vi "Actor Core.vi"(8 "error in":errorcluster, 11 "Island in":refnum<class "Island.lvclass">) -> (0 "error out":errorcluster, 3 "Actor out":refnum<class "Actor.lvclass">)   [LabVIEW 2018, in "Island Actor.lvlib" / "Island.lvclass"]
doc: "(<B>Filename</B>: Actor Framework.lvlib:Actor.lvclass:Actor Core.vi)\n\nReceives messages to the actor, reacts to them, and initiates any error handling that may shut the actor down.\n\nDescendant classes may override this VI to append parallel tasks for the actor to complete while it handles messages. Overrides use the Call Parent Method node."
uses:
  Island.lvclass
  C:/Users/Administrator/Desktop/LabVIEW EMS/EMS Generic Actor/EMS Generic/EMS Generic.lvclass
  C:/Users/Administrator/Desktop/LabVIEW EMS/Device Communication and Control Abstract Actor/Device Communication and Control Abstract/Device Communication and Control Abstract.lvclass
  C:/Users/Administrator/Desktop/LabVIEW EMS/Optimization/Generic Optimization Actor/Generic Optimization/Generic Optimization.lvclass
  <vilib>/ActorFramework/Actor/Actor.lvclass
  EMS Generic Actor/EMS Generic/EMS Generic.lvclass/EMS Generic.ctl
  <vilib>/ORNL/CSEISMIC DDS/CSEISMIC DDS Base/Data Types/DER_VF.ctl
  <vilib>/ORNL/CSEISMIC DDS/CSEISMIC DDS Base/Data Types/Controls/DeviceID.ctl
  <vilib>/ActorFramework/Actor/Actor.lvclass/Actor.ctl
  Device Communication and Control Abstract Actor/Device Communication and Control Abstract/Device Communication and Control Abstract.lvclass/Device Communication and Control Abstract.ctl
  Device Communication and Control Abstract Actor/Device Communication and Control Abstract Messages/Set DER VF Msg/Set DER VF Msg.lvclass/Set DER VF Msg.ctl
  <vilib>/ActorFramework/Message Enqueuer/Message Enqueuer.lvclass/Message Enqueuer.ctl
  Generic Optimization Actor/Generic Optimization/Optimization Controls/PCC Data.ctl
  <vilib>/ORNL/CSEISMIC DDS/CSEISMIC DDS Base/Data Types/SmartRelay_Measurement.ctl
  <vilib>/ORNL/CSEISMIC DDS/CSEISMIC DDS Base/Data Types/PCC_Transition.ctl
  Device Communication and Control Abstract Actor/Device Communication and Control Abstract Messages/Set PCC Transition Msg/Set PCC Transition Msg.lvclass/Set PCC Transition Msg.ctl
  Device Communication and Control Abstract Actor/Device Communication and Control Abstract Messages/Set DER VF Msg/Send Set DER VF.vi
  <vilib>/ActorFramework/Actor/Read Caller Enqueuer.vi
  Device Communication and Control Abstract Actor/Device Communication and Control Abstract Messages/Set PCC Transition Msg/Send Set PCC Transition.vi
  <vilib>/ActorFramework/Message Enqueuer/Enqueue.vi
  Device Communication and Control Abstract Actor/Device Communication and Control Abstract/Device Communication and Control Abstract.lvclass
  C:/Program Files (x86)/National Instruments/LabVIEW 2018/vi.lib/ActorFramework/Actor/Actor.lvclass
  Device Communication and Control Abstract Actor/Device Communication and Control Abstract Messages/Set DER VF Msg/Set DER VF Msg.lvclass
  C:/Program Files (x86)/National Instruments/LabVIEW 2018/vi.lib/ActorFramework/Message/Message.lvclass
  Device Communication and Control Abstract Actor/Device Communication and Control Abstract Messages/Set PCC Transition Msg/Set PCC Transition Msg.lvclass
  <vilib>/ActorFramework/Message Priority Queue/Priority Enqueue.vi
  Generic Optimization Actor/Generic Optimization/Generic Optimization.lvclass
  <vilib>/ORNL/CSEISMIC DDS/CSEISMIC DDS Base/CSEISMIC DDS.lvclass
  <vilib>/ORNL/CSEISMIC DDS/CSEISMIC DDS Base/Data Types/Controls/DeviceClass Selector.ctl
  <vilib>/ORNL/CSEISMIC DDS/CSEISMIC DDS Base/Data Types/DER_Control.ctl
  EMS Generic Actor/EMS Generic/EMS Generic.lvclass
  Utilities/Status Messaging.llb/Status Messaging.lvlib
panel:
  out "Solution Result":string="Waiting"
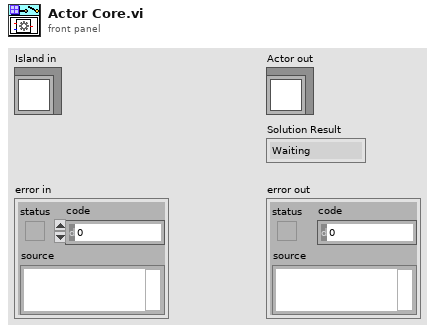
[diagram p1: front panel]
types:
  T1 = typedef "EMS Generic Actor.lvlib/EMS Generic.lvclass/Data Type DVRs.ctl" = cluster{"IED_Status":refnum<data-value>, "IED_Status_0":refnum<data-value>, "DER_Measurement":refnum<data-value>, "DER_Info":refnum<data-value>, "DER_Status":refnum<data-value>, "ES_Measurement":refnum<data-value>, "ES_Info":refnum<data-value>, "PV_Info":refnum<data-value>, "SmartRelay_Info":refnum<data-value>, "SmartRelay_Measurement":refnum<data-value>, "Meter_Info":refnum<data-value>, "Meter_Measurement":refnum<data-value>, "HVAC_Status":refnum<data-value>, "HVAC_Measurement":refnum<data-value>, "PriceData_RealTime":refnum<data-value>, "PriceData_Demand":refnum<data-value>, "PriceData_Energy":refnum<data-value>, "ForecastData_Long":refnum<data-value>, "ForecastData_Short":refnum<data-value>, "DER_Control":refnum<data-value>, "DER_SetPointF":refnum<data-value>, "DER_SetPointP":refnum<data-value>, "DER_SetPointQ":refnum<data-value>, "DER_SetPointPF":refnum<data-value>, "DER_SetPointV":refnum<data-value>, "PV_setCurtailment":refnum<data-value>, "PV_setRampRate":refnum<data-value>, "Relay_Control":refnum<data-value>, "Load_Control":refnum<data-value>, "HVAC_Control":refnum<data-value>, "Generator_Info":refnum<data-value>, "ForecastData_Long_Backup":refnum<data-value>, "PriceData_RealTime_Backup":refnum<data-value>}
  T2 = typedef "CSEISMIC DDS.lvlib/CSEISMIC DDS.lvclass/DER_VF.ctl" = cluster{"DeviceID":T3}
  T3 = typedef "CSEISMIC DDS.lvlib/CSEISMIC DDS.lvclass/DeviceID.ctl" = string
  T4 = typedef "CSEISMIC DDS.lvlib/CSEISMIC DDS.lvclass/DER_Control.ctl" = cluster{"DeviceID":T3, "Activate":bool, "Deactivate":bool}
  T5 = typedef "CSEISMIC DDS.lvlib/CSEISMIC DDS.lvclass/DeviceClass Selector.ctl" = u16
  T6 = typedef "EMS Generic Actor.lvlib/EMS Generic.lvclass/Global Configuration.ctl" = cluster{"Microgrid ID":u8, "VF Device ID":T3, "Ongrid VF Priority":T3[], "Offgrid VF Priority":T3[], "AutoSwap Offgrid VF":u32, "AutoSwap Offgrid VF Delay (sec)":dbl, "AutoSwap Resynch VF":u32, "PCC Device ID":T3, "Device ID Array":T3[], "Nominal Voltage":dbl, "Nominal Frequency":dbl, "Resynch Timeout (sec)":dbl, "Island VF Activate Timeout (sec)":dbl, "Island PCC Target Power (kW)":dbl, "Island PCC Target Power Timeout (sec)":dbl, "Island Grid Settle Time (sec)":dbl, "Island PCC Failure Timeout (sec)":dbl, "Activation Devices Present Timeout (sec)":dbl, "Activation Devices Activated Timeout (sec)":dbl, "Blackstart VF GenMode Wait (sec)":dbl, "Blackstart VF DERCtrl Wait (sec)":dbl, "Blackstart Success Wait (sec)":dbl, "OnGrid Optimization Delay (sec)":dbl, "OffGrid Optimization Delay (sec)":dbl, "Resynch Frequency (Hz)":dbl, "Optimization Path":string}
  T7 = typedef "Generic Optimization Actor.lvlib/Generic Optimization.lvclass/Bus by ID.ctl" = cluster{"DeviceID":T3, "Bus ID":dbl}
  T8 = typedef "Generic Optimization Actor.lvlib/Generic Optimization.lvclass/Electrical Network Optimization Data.ctl" = cluster{"From_Bus":dbl, "To_Bus":dbl, "Network Resistance":dbl, "Network Reactance":dbl, "Power Flow Limits":dbl[], "Linear Piecewise Power Flow":dbl[], "Reactive Flow Limit":dbl[], "Linear Piecewise Reactive Flow":dbl[]}
  T9 = typedef "CSEISMIC DDS.lvlib/CSEISMIC DDS.lvclass/SmartRelay_Measurement.ctl" = cluster{"DeviceID":T3, "PrimaryVoltage":dbl[], "SecondaryVoltage":dbl[], "Current":dbl[], "RealPower":dbl[], "ReactivePower":dbl[], "LineConfig":u8[], "Frequency":dbl}
  T10 = typedef "Generic Optimization Actor.lvlib/Generic Optimization.lvclass/PCC Data.ctl" = cluster{"PCC_max":dbl[], "PCC_min":dbl[], "QCC_max":dbl[], "QCC_min":dbl[]}
  T11 = typedef "CSEISMIC DDS.lvlib/CSEISMIC DDS.lvclass/IED_Status.ctl" = cluster{"DeviceID":T3, "Timestamp":T12, "MicrogridID":u8, "Active":bool, "Inactive":bool, "Error":i32, "Fault":bool, "ErrorString":string}
  T12 = typedef "CSEISMIC DDS.lvlib/CSEISMIC DDS.lvclass/Timestamp.ctl" = cluster{"Seconds":u64, "Remainder":u64}
  T13 = typedef "CSEISMIC DDS.lvlib/CSEISMIC DDS.lvclass/PCC_Transition.ctl" = cluster{"DeviceID":T3, "Island":bool, "Resynchronize":bool}
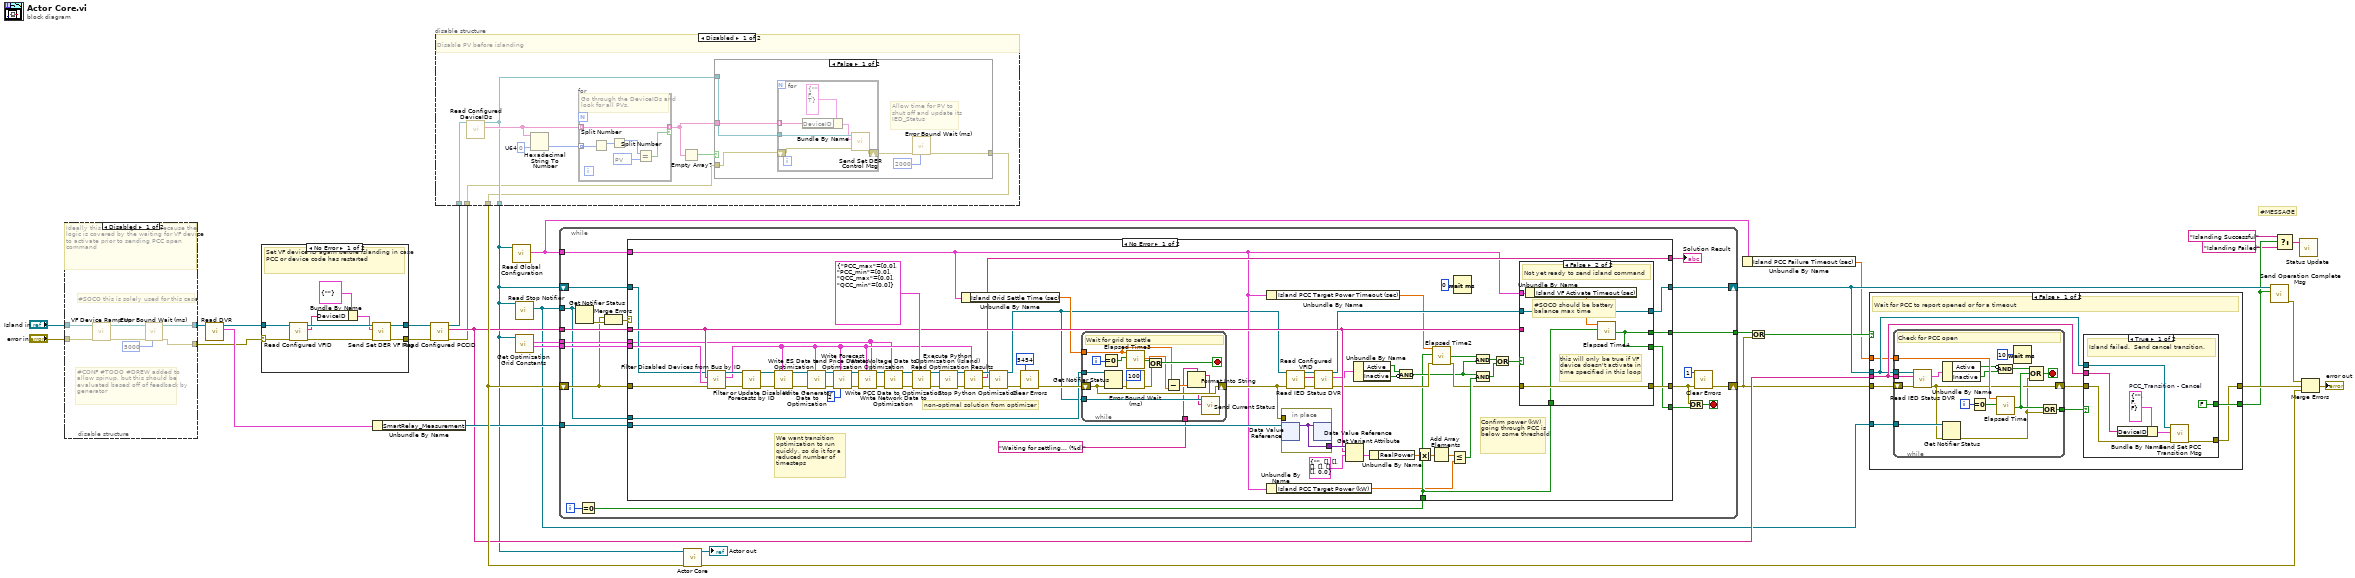
[diagram p0: block diagram]
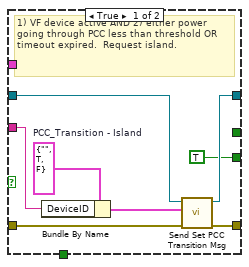
[diagram p4: hidden frame]
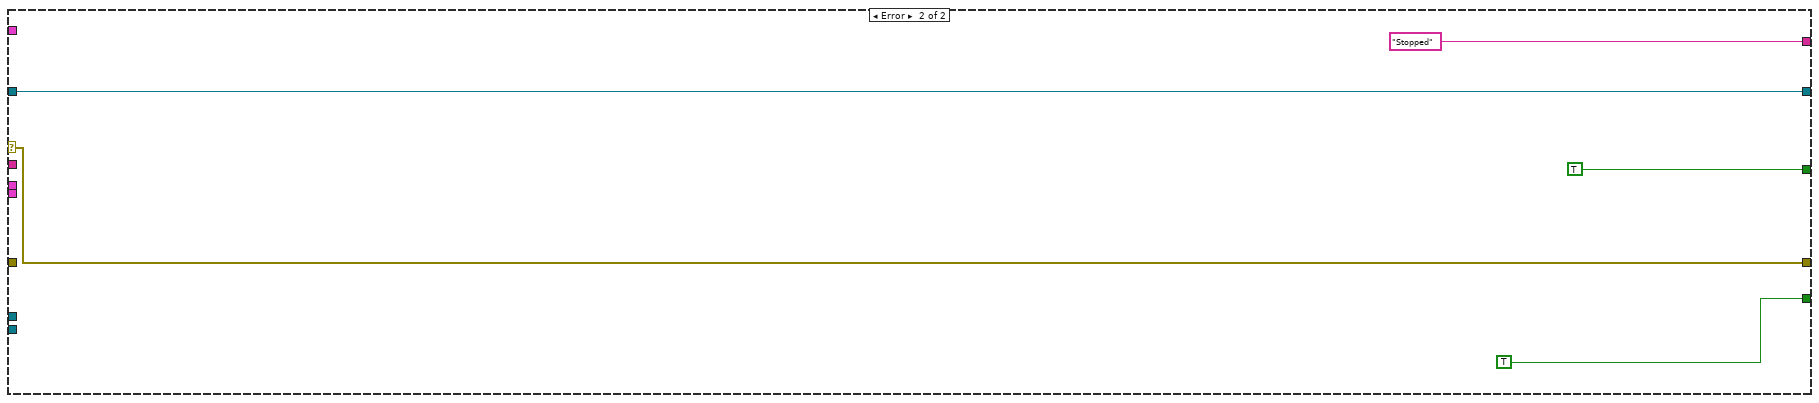
[diagram p5: hidden frame]
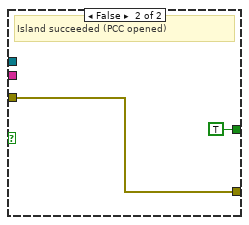
[diagram p8: hidden frame]
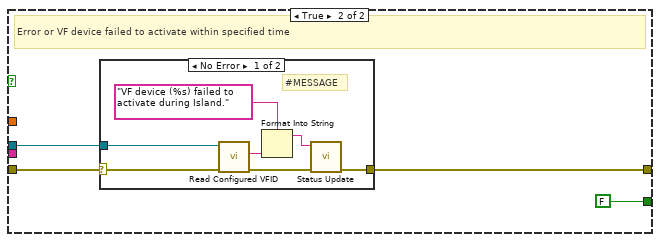
[diagram p9: hidden frame]
diagram:
  # "#MESSAGE"
  n1 = disable-structure shown="Disabled" {
    disable-tunnel: "Island in" -> [w38 w40]
    disable-tunnel: [w37 w40] -> w20
    disable-tunnel: "error in" -> [w36 w39]
    disable-tunnel: [w34 w39] -> w8
    frame Disabled {
      # "#SOCO this is solely used for this case"
      # "#CONF #TODO #DREW added to allow spinup, but this should be evaluated based off of feedback by generator"
      # "Ideally this is no longer used because the logic is covered by the waiting for VF device to activate prior to sending PCC open command"
      n2 = call "VF Device Ramp Up.vi"("error in"=w36, "Island in"=w38) -> ("error out"=w35:errorcluster, "Island out"=w37:refnum<class "Island.lvclass">)  [unwired: 8 in]
      n3 = call "Error Bound Wait (ms).vi"("milliseconds to wait (100)"=u32 5000 ("milliseconds to wait"), "error in"=w35) -> ("error out"=w34:errorcluster)  [unwired: 9 in]
    }
    frame Enabled {
    }
  }
  n4 = call "Read DVR.vi"("EMS Generic in"=w20) -> ("DVR"=w24:T1, "EMS Generic out"=w5:refnum<class "Island.lvclass">)  [unwired: 9 in]
  n5 = case shown="No Error" w8 {
    selector: w8 -> [w49 w51]
    tunnel: [w41 w51] -> w7
    tunnel: w5 -> [w48 w50]
    tunnel: [w44 w50] -> w6
    frame No Error {
      # "Set VF device ID again before islanding in case PCC or device code has restarted"
      n6 = call "Read Configured VFID.vi"("error in"=w49, "EMS Generic in"=w48) -> ("error out"=w46:errorcluster, "VFID"=w43:T3, "EMS Generic out"=w45:refnum<class "Island.lvclass">)  [unwired: 7 in]
      n7 = Bundle By Name(cluster=T2 {"DeviceID"=""} ("DER_VF"), "DeviceID"=w43) -> (w42:T2)
      n8 = call "Send Set DER VF Msg.vi"("error in"=w46, "DER_VF"=w42, "SCADA Sub Abstract in"=w45) -> ("error out"=w41:errorcluster, "dup SCADA Sub Abstract"=w44:refnum<class "Island.lvclass">)  [unwired: 7 in]
    }
    frame Error {
    }
  }
  n9 = Unbundle By Name(w24) -> ("SmartRelay_Measurement"=w23:refnum<data-value>)
  n10 = call "Read Configured PCCID.vi"("error in"=w7, "EMS Generic in"=w6) -> ("error out"=w16:errorcluster, "PCCID"=w22:T3, "EMS Generic out"=w26:refnum<class "Island.lvclass">)  [unwired: 7 in]
  n11 = disable-structure shown="Disabled" {
    disable-tunnel: w26 -> [w55 w80]
    disable-tunnel: [w54 w80] -> w11
    disable-tunnel: w16 -> [w53 w81]
    disable-tunnel: [w52 w81] -> w28
    frame Disabled {
      w60 = u64 0  # U64
      # "Disable PV before islanding"
      n12 = call "Read Configured DeviceIDs.vi"("EMS Generic in"=w55) -> ("DeviceIDs"=w59:T3[], "EMS Generic out"=w54:refnum<class "Island.lvclass">)  [unwired: 8 in, 1 out]
      n13 = Hexadecimal String To Number(string=w59, default (0uL)=w60) -> (number=w58:u64[])  [unwired: 1 in, 1 out]
      n14 = for {
        tunnel: w59 -> [w78] mode=indexing
        tunnel: [w78] -> w56 mode=indexing if=w75
        tunnel: w58 -> [w74] mode=indexing
        w77 = T5 514 items=["Invalid"=0, "IED"=256, "DER"=512, "Relay"=768, "Meter"=1024, "Load"=1280, "Energy Storage"=513, "PV"=514, "Generator"=515, "Smart Relay"=769, "PCC"=770, "Smart Meter"=1025, "PMU"=1026, "HVAC"=1281] ("DeviceClass")
        # "Go through the DeviceIDs and look for all PVs."
        n15 = Split Number(x=w74) -> (hi(x)=w79:u32)  [unwired: 1 out]
        n16 = Split Number(x=w79) -> (hi(x)=w76:u16)  [unwired: 1 out]
        n17 = Equal?(x=w76, y=w77) -> (x = y?=w75:bool)
      }
      n18 = Empty Array?(array=w56) -> (empty?=w57:bool)
      n19 = case shown="False" w57 {
        tunnel: w56 -> [w66 _]
        tunnel: w54 -> [w64 _]
        tunnel: [w62 w73] -> w52
        tunnel: w53 -> [w65 w73]
        frame False {
          # "Allow time for PV to shut off and update its IED_Status"
          n20 = for {
            tunnel: w66 -> [w72] mode=indexing
            tunnel: w64 -> [w70]
            shift-right: [w67] -> w63
            shift-left: w65 -> [w68]
            n21 = Bundle By Name(cluster=T4 {"DeviceID"="", "Activate"=FALSE, "Deactivate"=TRUE} ("DER_Control"), "DeviceID"=w72) -> (w69:T4)
            n22 = call "Send Set DER Control Msg.vi"("error in"=w68, "DER_Control"=w69, "SCADA Sub Abstract in"=w70) -> ("error out"=w67:errorcluster)  [unwired: 7 in, 1 out]
          }
          n23 = call "Error Bound Wait (ms).vi"("milliseconds to wait (100)"=u32 2000 ("milliseconds to wait"), "error in"=w63) -> ("error out"=w62:errorcluster)  [unwired: 9 in]
        }
        frame True {
        }
      }
    }
    frame Enabled {
    }
  }
  n24 = call "Read Global Configuration.vi"("EMS Generic in"=w11) -> ("Global Configuration"=w10:T6)  [unwired: 8 in, 2 out]
  n25 = call "Read Stop Notifier.vi"("EMS Generic in"=w11) -> ("stop"=w15:refnum<notifier>)  [unwired: 9 in, 1 out]
  n26 = call "Get Optimization Grid Constants.vi"("Generic Optimization in"=w11) -> ("Bus by ID"=w27:T7[], "Network Data"=w30:T8[])  [unwired: 8 in, 1 out]
  n27 = while {
    tunnel: w30 -> [w101]
    tunnel: w27 -> [w99]
    tunnel: w23 -> [w98]
    tunnel: w22 -> [w97]
    shift-right: [w90] -> w14
    shift-left: w28 -> [w94]
    shift-right: [w100] -> w19
    shift-left: w11 -> [w96]
    tunnel: w15 -> [w86]
    tunnel: [w83] -> w13
    tunnel: w10 -> [w82]
    i -> [w85]
    stop <- w87 stop-if-true
    n28 = Get Notifier Status(notifier=w86) -> (error out=w95:errorcluster)  [unwired: 1 in, 4 out]
    n29 = Equal To 0?(x=w85) -> (x = 0?=w84:bool)
    n30 = Merge Errors(w94, w95) -> (w93:errorcluster)
    n31 = case shown="No Error" w93 {
      selector: w93 -> [_ w202]
      tunnel: w101 -> [w104 _]
      tunnel: [w161 w202] -> w89
      tunnel: [w160 w203] -> w100
      tunnel: w94 -> [w154 _]
      tunnel: w99 -> [w153 _]
      tunnel: w98 -> [w142 _]
      tunnel: w97 -> [w136 _]
      tunnel: w96 -> [w135 w203]
      tunnel: [w133 "Stopped" ("Solution Result")] -> w92
      tunnel: [w111 TRUE] -> w88
      tunnel: w86 -> [w129 _]
      tunnel: w84 -> [w110 _]
      tunnel: [w109 TRUE ("Time has Elapsed")] -> w83
      tunnel: w82 -> [w105 _]
      frame No Error {
        # "Confirm power (kW) going through PCC is below some threshold"
        # "We want transition optimization to run quickly, so do it for a reduced number of timesteps"
        # "non-optimal solution from optimizer"
        n32 = call "Filter Disabled Devices from Bus by ID.vi"("error in"=w154, "BusData"=w153, "PCCID"=w136, "Generic Optimization in"=w135) -> ("dup error out"=w152:errorcluster, "Filtered Bus by ID"=w148:T7[], "Generic Optimization out"=w150:refnum<class "Island.lvclass">)  [unwired: 5 in]
        n33 = call "Filter or Update Disabled Forecasts by ID.vi"("error in"=w152, "Generic Optimization in"=w150) -> ("dup error out"=w151:errorcluster, "Generic Optimization out"=w149:refnum<class "Island.lvclass">)  [unwired: 8 in]
        n34 = call "Write ES Data to Optimization.vi"("Bus by ID"=w148, "error in"=w151, "Generic Optimization in"=w149) -> ("error out"=w168:errorcluster, "Generic Optimization out"=w167:refnum<class "Island.lvclass">)  [unwired: 7 in]
        n35 = call "Write Generator Data to Optimization.vi"("Bus by ID"=w148, "error in"=w168, "Generic Optimization in"=w167) -> ("error out"=w147:errorcluster, "Generic Optimization out"=w145:refnum<class "Island.lvclass">)  [unwired: 7 in]
        n36 = call "Write Forecast and Price Data to Optimization.vi"("Max Forecast Length (-1: no limit)"=2, "Bus by ID"=w148, "error in"=w147, "Generic Optimization in"=w145) -> ("error out"=w146:errorcluster, "Generic Optimization out"=w144:refnum<class "Island.lvclass">)  [unwired: 6 in]
        n37 = call "Write Voltage Data to Optimization.vi"("Network Data Array"=w104, "Bus by ID"=w148, "error in"=w146, "Generic Optimization in"=w144) -> ("error out"=w169:errorcluster, "Generic Optimization out"=w166:refnum<class "Island.lvclass">)  [unwired: 6 in]
        n38 = call "Write Network Data to Optimization.vi"("Network Data Array"=w104, "error in"=w169, "Generic Optimization in"=w166) -> ("error out"=w158:errorcluster, "Generic Optimization out"=w159:refnum<class "Island.lvclass">)  [unwired: 7 in]
        n39 = call "Write PCC Data to Optimization.vi"("PCC Data"=T10 {"PCC_max"=[0.0], "PCC_min"=[0.0], "QCC_max"=[0.0], "QCC_min"=[0.0]}, "error in"=w158, "Generic Optimization in"=w159) -> ("error out"=w157:errorcluster, "Generic Optimization out"=w156:refnum<class "Island.lvclass">)  [unwired: 7 in]
        n40 = call "Execute Python Optimization (Island).vi"("error in"=w157, "Island in"=w156) -> ("error out"=w164:errorcluster, "Island out"=w165:refnum<class "Island.lvclass">)  [unwired: 8 in]
        n41 = Unbundle By Name(w105) -> ("Island Grid Settle Time (sec)"=w108:dbl)
        n42 = call "Read Optimization Results.vi"("Bus by ID Array"=w148, "error in"=w164, "Generic Optimization in"=w165) -> ("error out"=w162:errorcluster, "Solution Result"=w133:string, "Generic Optimization out"=w163:refnum<class "Island.lvclass">)  [unwired: 6 in]
        n43 = call "Stop Python Optimization.vi"("error in"=w162, "Generic Optimization in"=w163) -> ("error out"=w131:errorcluster, "Generic Optimization out"=w103:refnum<class "Island.lvclass">)  [unwired: 8 in]
        n44 = call <vilib>:"Clear Errors.vi"("error in (no error)"=w131, "specific error code to clear (0: all)"=5454) -> ("error out"=w130:errorcluster)  [unwired: 4 in, 1 out]
        n45 = while {
          shift-right: [w178] -> w126
          shift-left: w130 -> [w178]
          tunnel: w129 -> [w180]
          tunnel: w108 -> [w174]
          tunnel: w103 -> [w177]
          tunnel: "Waiting for settling... (%d)" ("Current Status") -> [w171]
          i -> [w183]
          stop <- w181 stop-if-true
          # "Wait for grid to settle"
          n46 = Equal To 0?(x=w183) -> (x = 0?=w184:bool)
          n47 = Get Notifier Status(notifier=w180, error in (no error)=w178) -> (error out=w179:errorcluster)  [unwired: 4 out]
          n48 = call "Error Bound Wait (ms).vi"("milliseconds to wait (100)"=u32 100 ("milliseconds to wait"), "error in"=w179) -> ("error out"=w176:errorcluster)  [unwired: 9 in]
          n49 = call "Elapsed Time3"("Time Target (s)"=w174, "Reset"=w184) -> ("Elapsed Time (s)"=w173:dbl, "Time has Elapsed"=w182:bool)  [unwired: 10 in, 6 out]
          n50 = Or(x=w182, y=w176) -> (x .or. y?=w181:bool)
          n51 = Subtract(x=w174, y=w173) -> (x-y=w172:dbl)
          n52 = Format Into String(format string=w171, w172) -> (resulting string=w170:string)  [unwired: 2 in, 1 out]
          n53 = call "Send Current Status.vi"("Current Status"=w170, "Device Communication and Control Abstract in"=w177) -> ()  [unwired: 8 in, 2 out]
        }
        n54 = Unbundle By Name(w105) -> ("Island PCC Target Power Timeout (sec)"=w107:dbl)
        n55 = Unbundle By Name(w105) -> ("Island PCC Target Power (kW)"=w106:dbl)
        n56 = in-place {
          in-place-border: [w199] -> w141
          in-place-border: w126 -> [_]
          n57 = in-place-dvr #1(w142) -> (w199:variant)  [unwired: 1 out]
          n58 = in-place-dvr #1(w199) -> ()  [unwired: 2 out]
        }
        n59 = call "Read Configured VFID.vi"("error in"=w126, "EMS Generic in"=w103) -> ("error out"=w125:errorcluster, "VFID"=w123:T3, "EMS Generic out"=w124:refnum<class "Island.lvclass">)  [unwired: 7 in]
        n60 = call "Read IED Status DVR.vi"("error in"=w125, "DeviceID"=w123, "EMS Generic in"=w124) -> ("error out"=w119:errorcluster, "IED_Status"=w122:T11, "EMS Generic out"=w127:refnum<class "Island.lvclass">)  [unwired: 5 in, 1 out]
        n61 = Get Variant Attribute(Variant=w141, name=w136, default value (empty Variant)=T9 {"DeviceID"="", "PrimaryVoltage"=[], "SecondaryVoltage"=[], "Current"=[], "RealPower"=[], "ReactivePower"=[], "LineConfig"=[], "Frequency"=0.0} ("SmartRelay_Measurement")) -> (value=w139:T9)  [unwired: 1 in, 3 out]
        n62 = Unbundle By Name(w122) -> ("Active"=w121:bool, "Inactive"=w120:bool)
        n63 = Unbundle By Name(w139) -> ("RealPower"=w138:dbl[])
        n64 = Compound Arithmetic op=AND(w121, invert w120) -> (w114:bool)
        n65 = Absolute Value(x=w138) -> (abs(x)=w117:dbl[])
        n66 = call "Elapsed Time2"("Time Target (s)"=w107, "Reset"=w110, "error in (no error)"=w119) -> ("Time has Elapsed"=w115:bool, "error out"=w118:errorcluster)  [unwired: 9 in, 6 out]
        n67 = Add Array Elements(numeric array=w117) -> (sum=w137:dbl)
        n68 = Less Or Equal?(x=w137, y=w106) -> (x <= y?=w128:bool)
        n69 = Wait (ms)(milliseconds to wait=u32 0) -> ()  [unwired: 1 out]
        n70 = Compound Arithmetic op=AND(w115, w114) -> (w113:bool)
        n71 = Compound Arithmetic op=AND(w114, w128) -> (w116:bool)
        n72 = Or(x=w113, y=w116) -> (x .or. y?=w112:bool)
        n73 = case shown="False" w112 {
          tunnel: w127 -> [w192 w198]
          tunnel: w118 -> [w188 w197]
          tunnel: [w187 w197] -> w161
          tunnel: [w191 w198] -> w160
          tunnel: w136 -> [w189 _]
          tunnel: [TRUE w195] -> w111
          tunnel: w110 -> [_ w196]
          tunnel: [_ w195] -> w109
          tunnel: w105 -> [_ w194]
          frame True {
            w190 = T13 {"DeviceID"="", "Island"=TRUE, "Resynchronize"=FALSE}  # PCC_Transition - Island
            # "1) VF device active AND 2) either power going through PCC less than threshold OR timeout expired.  Request island."
            n74 = Bundle By Name(cluster=w190, "DeviceID"=w189) -> (w186:T13)
            n75 = call "Send Set PCC Transition Msg.vi"("error in"=w188, "PCC_Transition"=w186, "SCADA Sub Abstract in"=w192) -> ("error out"=w187:errorcluster, "dup SCADA Sub Abstract"=w191:refnum<class "Island.lvclass">)  [unwired: 7 in]
          }
          frame False {
            # "#SOCO should be battery balance max time"
            # "this will only be true if VF device doesn't activate in time specified in this loop"
            # "Not yet ready to send island command"
            n76 = Unbundle By Name(w194) -> ("Island VF Activate Timeout (sec)"=w193:dbl)
            n77 = call "Elapsed Time4"("Time Target (s)"=w193, "Reset"=w196) -> ("Time has Elapsed"=w195:bool)  [unwired: 10 in, 7 out]
          }
        }
      }
      frame Error {
      }
    }
    "Solution Result" <- w92
    n78 = Or(x=w89, y=w88) -> (x .or. y?=w87:bool)
    n79 = call <vilib>:"Clear Errors.vi"("error in (no error)"=w89, "specific error code to clear (0: all)"=1) -> ("error out"=w90:errorcluster)  [unwired: 4 in, 1 out]
  }
  n80 = call-parent "Actor Core.vi"("error in"=w28, "Actor in"=w11) -> ("error out"=w32:errorcluster, "Actor out"=→"Actor out":refnum<class "Actor.lvclass">)  [unwired: 8 in]
  n81 = Unbundle By Name(w10) -> ("Island PCC Failure Timeout (sec)"=w9:dbl)
  n82 = Or(x=w13, y=w14) -> (x .or. y?=w12:bool)
  n83 = case shown="False" w12 {
    tunnel: [w206 w241] -> w25
    tunnel: w19 -> [w207 w240]
    tunnel: w22 -> [w208 _]
    tunnel: [w211 FALSE ("Time has Elapsed")] -> w4
    tunnel: w15 -> [w212 _]
    tunnel: w14 -> [w213 w242]
    tunnel: w9 -> [w205 _]
    frame False {
      # "Wait for PCC to report opened or for a timeout"
      n84 = while {
        tunnel: w207 -> [w235]
        tunnel: w208 -> [w234]
        shift-right: [w227] -> w209
        shift-left: w213 -> [w232]
        tunnel: w212 -> [w231]
        tunnel: [w229] -> w210
        tunnel: w205 -> [w228]
        i -> [w237]
        stop <- w239 stop-if-true
        # "Check for PCC open"
        n85 = call "Read IED Status DVR.vi"("error in"=w232, "DeviceID"=w234, "EMS Generic in"=w235) -> ("error out"=w227:errorcluster, "IED_Status"=w233:T11)  [unwired: 5 in, 2 out]
        n86 = Unbundle By Name(w233) -> ("Active"=w225:bool, "Inactive"=w224:bool)
        n87 = Get Notifier Status(notifier=w231, error in (no error)=w227) -> (error out=w226:errorcluster)  [unwired: 4 out]
        n88 = Equal To 0?(x=w237) -> (x = 0?=w236:bool)
        n89 = call "Elapsed Time"("Time Target (s)"=w228, "Reset"=w236) -> ("Time has Elapsed"=w230:bool)  [unwired: 10 in, 7 out]
        n90 = Compound Arithmetic op=AND(invert w225, w224) -> (w223:bool)
        n91 = Wait (ms)(milliseconds to wait=u32 10) -> ()  [unwired: 1 out]
        n92 = Compound Arithmetic op=OR(w223, w230, w226) -> (w239:bool)
        n93 = Or(x=w230, y=w226) -> (x .or. y?=w229:bool)
      }
      n94 = case shown="True" w210 {
        tunnel: w207 -> [w220 _]
        tunnel: w209 -> [w217 w222]
        tunnel: [w216 w222] -> w206
        tunnel: w208 -> [w218 _]
        tunnel: [FALSE TRUE] -> w211
        frame True {
          w219 = T13 {"DeviceID"="", "Island"=FALSE, "Resynchronize"=FALSE}  # PCC_Transition - Cancel
          # "Island failed.  Send cancel transition."
          n95 = Bundle By Name(cluster=w219, "DeviceID"=w218) -> (w215:T13)
          n96 = call "Send Set PCC Transition Msg.vi"("error in"=w217, "PCC_Transition"=w215, "SCADA Sub Abstract in"=w220) -> ("error out"=w216:errorcluster)  [unwired: 7 in, 1 out]
        }
        frame False {
          # "Island succeeded (PCC opened)"
        }
      }
    }
    frame True {
      # "Error or VF device failed to activate within specified time"
      n97 = case shown="No Error" w242 {
        selector: w242 -> [w249 w251]
        tunnel: [w250 w251] -> w241
        tunnel: w240 -> [w244 _]
        frame No Error {
          # "#MESSAGE"
          n98 = call "Read Configured VFID.vi"("error in"=w249, "EMS Generic in"=w244) -> ("error out"=w248:errorcluster, "VFID"=w247:T3)  [unwired: 7 in, 1 out]
          n99 = Format Into String(format string="VF device (%s) failed to activate during Island.", w247) -> (resulting string=w245:string)  [unwired: 2 in, 1 out]
          n100 = call "Status Update.vi"("error in"=w248, "Status Update"=w245) -> ("error out"=w250:errorcluster)  [unwired: 8 in, 1 out]
        }
        frame Error {
        }
      }
    }
  }
  n101 = call "Send Operation Complete Msg.vi"("Operation Complete"=w4, "Generic Optimization in"=w19) -> ("error out"=w18:errorcluster)  [unwired: 8 in, 1 out]
  n102 = Select(t="Islanding Successful", s=w4, f="Islanding Failed") -> (s? t:f=w1:string)
  n103 = call "Status Update.vi"("Status Update"=w1) -> ()  [unwired: 9 in, 2 out]
  n104 = Merge Errors(w18, w25, w32) -> (→"error out":errorcluster)
